vi "Asylum_Driver_StartXYPISLoops.vi"(8 "error in (no error)":errorcluster, 9 "Y PIS Controls":T1, 10 "X PIS Controls":T1, 11 "Application":refnum<k7>) -> (0 "error out":errorcluster, 3 "Application":refnum<k7>)   [LabVIEW 2019]
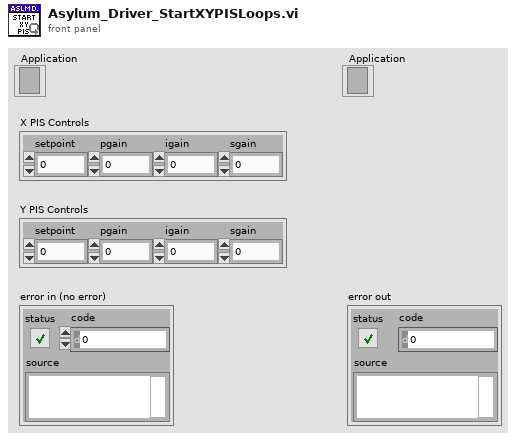
[diagram p1: front panel]
types:
  T1 = cluster{"setpoint":dbl, "pgain":dbl, "igain":dbl, "sgain":dbl}
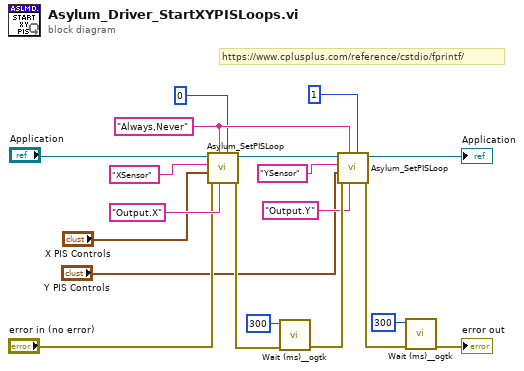
[diagram p0: block diagram]
diagram:
  w16 = "Always,Never" ("eventString")
  # "https://www.cplusplus.com/reference/cstdio/fprintf/"
  n1 = call <userlib>:"Asylum_SetPISLoop.vi"("whichLoop"=0, "outChannelString"="Output.X", "eventString"=w16, "error in (no error)"="error in (no error)", "PIS Controls"="X PIS Controls", "inChannelString"="XSensor", "Application"="Application") -> ("error out"=w18:errorcluster, "Application"=w11:refnum<k7>)  [unwired: 3 in]
  n2 = call <userlib>:"Wait (ms)__ogtk.vi"("error in (no error)"=w18, "milliseconds to wait"=u32 300) -> ("error out"=w19:errorcluster)  [unwired: 8 in, 1 out]
  n3 = call <userlib>:"Asylum_SetPISLoop.vi"("whichLoop"=1, "outChannelString"="Output.Y", "eventString"=w16, "error in (no error)"=w19, "PIS Controls"="Y PIS Controls", "inChannelString"="YSensor", "Application"=w11) -> ("error out"=w5:errorcluster, "Application"=→"Application":refnum<k7>)  [unwired: 3 in]
  n4 = call <userlib>:"Wait (ms)__ogtk.vi"("error in (no error)"=w5, "milliseconds to wait"=u32 300) -> ("error out"=→"error out":errorcluster)  [unwired: 8 in, 1 out]
